vi "摆角通道.vi"() -> (0 "error out":errorcluster caption="错误输出", 1 "task out":refnum<k21> caption="任务输出")   [LabVIEW 2015]
uses:
  <vilib>/DAQmx/create/channels.llb/DAQmx Create Channel (CI-Count Edges).vi
  <resource>/objmgr/daqmx.rc
panel:
  in  "数值":u32=1
  in  "DAQmx设备名":tag="Dev3"
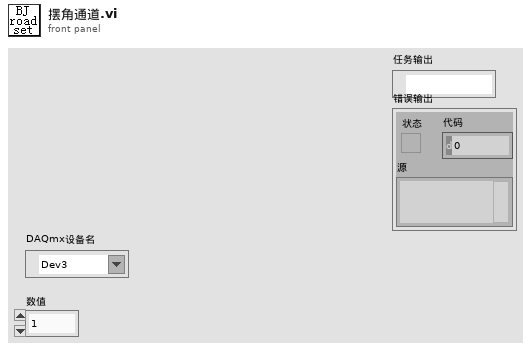
[diagram p1: front panel]
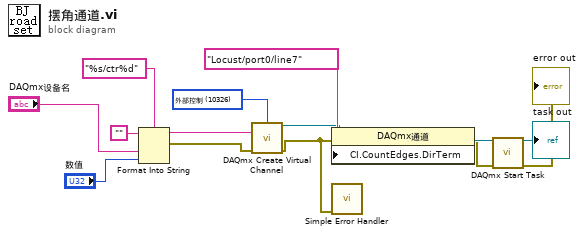
[diagram p0: block diagram]
diagram:
  w10 = 10326 items=["升值计数"=10128, "减值计数"=10124, "外部控制"=10326] ("count direction")
  n1 = Format Into String(format string="%s/ctr%d" ("格式字符串"), initial string="" ("初始字符串"), "DAQmx设备名", "数值") -> (resulting string=w4:string, error out=w9:errorcluster)  [unwired: 1 in]
  n2 = call-poly <vilib>:"DAQmx Create Virtual Channel.vi"("count direction"=w10, "counter"=w4, "error in"=w9) -> ("task out"=w7:refnum<k21>, "error out"=w3:errorcluster)  [unwired: 11 in]
  n3 = property class="DAQmx通道"(reference=w7, error in=w3, "CI.CountEdges.DirTerm"=tag "Locust/port0/line7" ("CI.CountEdges.Term")) -> (reference out=w6:refnum<k21>, error out=w5:errorcluster)
  n4 = call <vilib>:"Simple Error Handler.vi"("error in (no error)"=w3) -> ()  [unwired: 4 in, 5 out]
  n5 = call <vilib>:"DAQmx Start Task.vi"("task/channels in"=w6, "error in"=w5) -> ("task out"=→"task out":refnum<k21>, "error out"=→"error out":errorcluster)  [unwired: 12 in]
